vi "insert or remove.vi"(6 "replace entry if exists":bool, 7 "action":T5, 8 "error in (no error)":errorcluster, 10 "entry":T1, 11 "id":string) -> (0 "error out":errorcluster)   [LabVIEW 2024, in "controls manager.lvlib"]
uses:
  controls manager.lvlib
  insert or remove.ctl
  entry type.ctl
  control.ctl
  controls plan.ctl
  key value pair.ctl
  fgv actions.ctl
  <vilib>/Utility/error.llb/Error Cluster From Error Code.vi
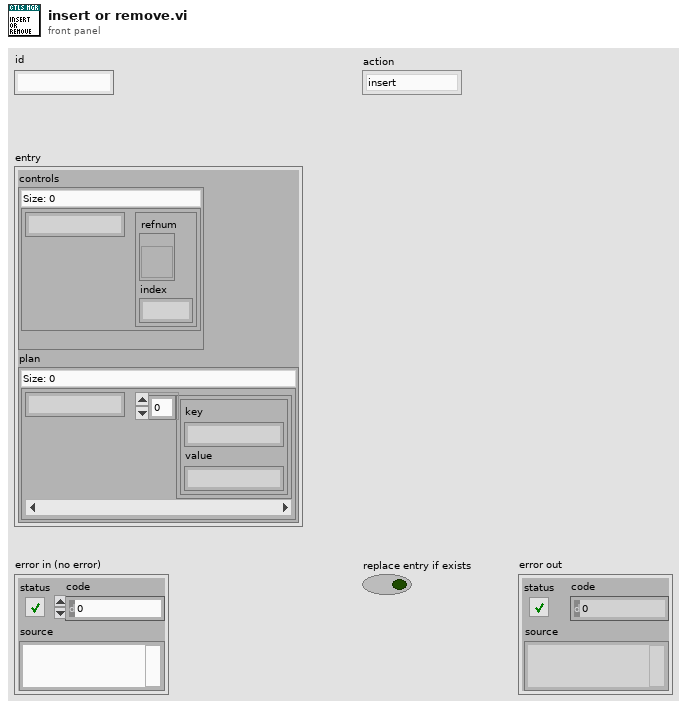
[diagram p1: front panel]
types:
  T1 = typedef "controls manager.lvlib/entry type.ctl" = cluster{"controls":map{string, T2}, "plan":T3}
  T2 = typedef "controls manager.lvlib/control.ctl" = cluster{"refnum":refnum<vi>, "index":i32}
  T3 = typedef "controls manager.lvlib/controls plan.ctl" = map{string, T4[]}
  T4 = typedef "controls manager.lvlib/key value pair.ctl" = cluster{"key":string, "value":string}
  T5 = typedef "controls manager.lvlib/insert or remove.ctl" = enum16{"insert", "remove"}
  T6 = typedef "controls manager.lvlib/fgv actions.ctl" = enum16{"create", "get", "destroy"}
  T7 = typedef "controls manager.lvlib/collection type.ctl" = map{string, T1}
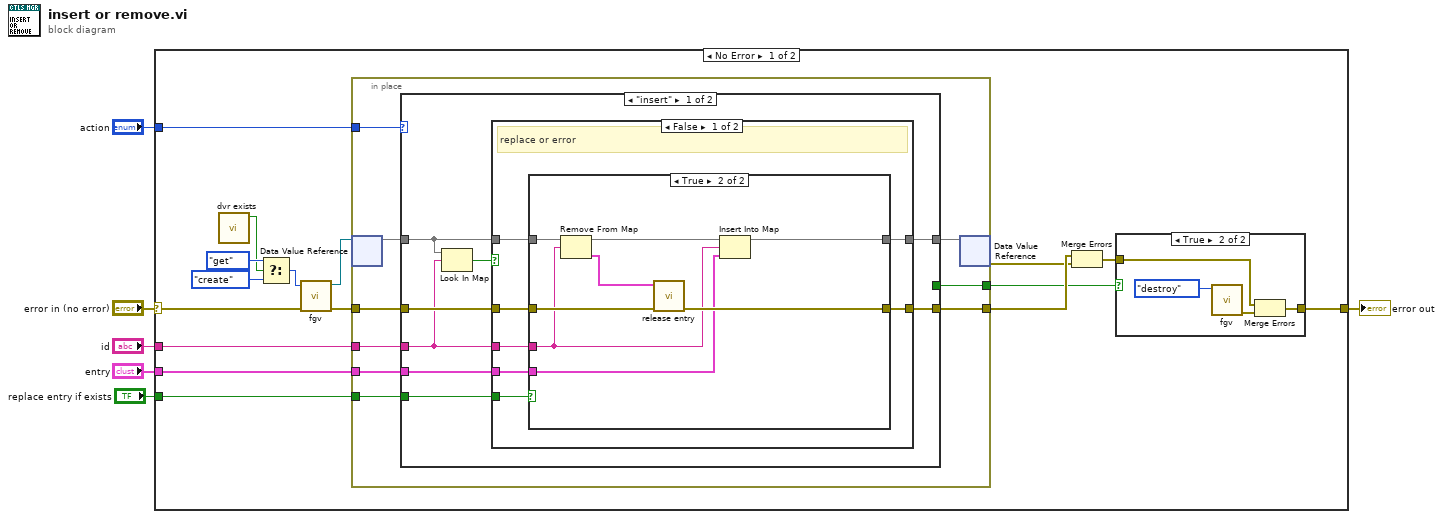
[diagram p0: block diagram]
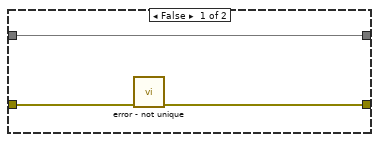
[diagram p2: hidden frame]
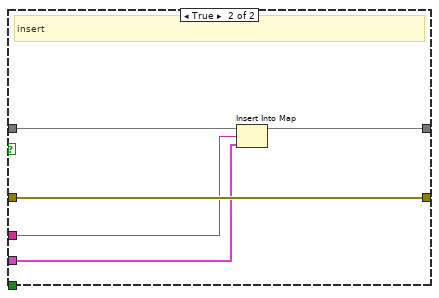
[diagram p3: hidden frame]
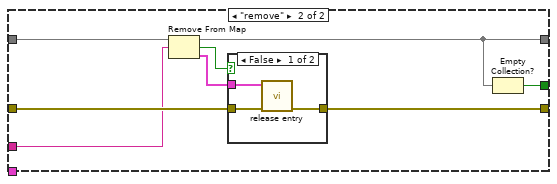
[diagram p4: hidden frame]
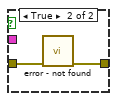
[diagram p5: hidden frame]
diagram:
  n1 = case shown="No Error" "error in (no error)" {
    selector: "error in (no error)" -> [w10 w81]
    tunnel: "replace entry if exists" -> [w22 _]
    tunnel: [w18 w81] -> w4
    tunnel: "entry" -> [w12 _]
    tunnel: "action" -> [w17 _]
    tunnel: "id" -> [w11 _]
    frame No Error {
      n2 = call "dvr exists.vi"() -> ("exists"=w7:bool)  [unwired: 10 in, 1 out]
      n3 = Select(t=fgv_actions."get", s=w7, f=fgv_actions."create") -> (s? t:f=w14:T6)
      n4 = call "fgv.vi"("error in (no error)"=w10, "action"=w14) -> ("error out"=w9:errorcluster, "dvr"=w16:refnum<data-value>)  [unwired: 8 in]
      n5 = in-place {
        in-place-border: [w29] -> w8
        in-place-border: w12 -> [w28]
        in-place-border: w22 -> [w27]
        in-place-border: w9 -> [w26]
        in-place-border: [w25] -> w21
        in-place-border: w11 -> [w24]
        in-place-border: w17 -> [w23]
        n6 = in-place-dvr #1(w16) -> (w31:T7)  [unwired: 1 out]
        n7 = case shown="\"insert\"" w23 {
          tunnel: w31 -> [w33 w65]
          tunnel: [w32 w64] -> w30
          tunnel: [_ w70] -> w29
          tunnel: w28 -> [w39 _]
          tunnel: w27 -> [w38 _]
          tunnel: w26 -> [w37 w69]
          tunnel: [w36 w68] -> w25
          tunnel: w24 -> [w35 w63]
          frame "insert" {
            n8 = Look In Map(map=w33, key=w35) -> (key not found?=w34:bool)  [unwired: 1 in, 1 out]
            n9 = case shown="False" w34 {
              tunnel: [w43 w61] -> w32
              tunnel: w33 -> [w45 w60]
              tunnel: w39 -> [w44 w59]
              tunnel: w38 -> [w46 _]
              tunnel: w37 -> [w42 w62]
              tunnel: [w41 w62] -> w36
              tunnel: w35 -> [w40 w58]
              frame False {
                # "replace or error"
                n10 = case shown="True" w46 {
                  tunnel: w45 -> [w49 w56]
                  tunnel: w44 -> [_ w53]
                  tunnel: [w49 w52] -> w43
                  tunnel: w42 -> [w48 w51]
                  tunnel: [w47 w57] -> w41
                  tunnel: w40 -> [_ w50]
                  frame False {
                    n11 = call "error - not unique.vi"("error in (no error)"=w48) -> ("error out"=w47:errorcluster)  [unwired: 10 in]
                  }
                  frame True {
                    n12 = Remove From Map(10:w50, 11:w56) -> (1:w55:T1, 3:w54:T7)  [unwired: 1 out]
                    n13 = call "release entry.vi"("error in (no error)"=w51, "entry"=w55) -> ("error out"=w57:errorcluster)  [unwired: 9 in]
                    n14 = Insert Into Map(map in=w54, key=w50, value=w53) -> (map out=w52:T7)  [unwired: 2 out]
                  }
                }
              }
              frame True {
                # "insert"
                n15 = Insert Into Map(map in=w60, key=w58, value=w59) -> (map out=w61:T7)  [unwired: 2 out]
              }
            }
          }
          frame "remove" {
            n16 = Remove From Map(10:w63, 11:w65) -> (1:w67:T1, 2:w66:bool, 3:w64:T7)
            n17 = case shown="False" w66 {
              tunnel: w67 -> [w73 _]
              tunnel: w69 -> [w72 w75]
              tunnel: [w71 w74] -> w68
              frame False {
                n18 = call "release entry.vi"("error in (no error)"=w72, "entry"=w73) -> ("error out"=w71:errorcluster)  [unwired: 9 in]
              }
              frame True {
                n19 = call "error - not found.vi"("error in (no error)"=w75) -> ("error out"=w74:errorcluster)  [unwired: 10 in]
              }
            }
            n20 = Empty Collection?(1:w64) -> (0:w70:bool)
          }
        }
        n21 = in-place-dvr #1(w30) -> (w20:errorcluster)  [unwired: 1 out]
      }
      n22 = Merge Errors(w21, w20) -> (w19:errorcluster)
      n23 = case shown="True" w8 {
        tunnel: w19 -> [w76 w79]
        tunnel: [w76 w80] -> w18
        frame False {
        }
        frame True {
          n24 = call "fgv.vi"("action"=fgv_actions."destroy") -> ("error out"=w77:errorcluster)  [unwired: 9 in, 1 out]
          n25 = Merge Errors(w79, w77) -> (w80:errorcluster)
        }
      }
    }
    frame Error {
    }
  }
  "error out" <- w4
